vi "NI VeriStand - Close Workspace Window.vi"(8 "error in (no error)":errorcluster, 11 "Project Ref in":T1) -> (0 "error out":errorcluster, 3 "Project Ref out":T1)   [LabVIEW 2020, in "NI_VS Project ExecutionAPI.lvlib"]
doc: "Closes the <B>Workspace</B> window for an NI VeriStand project."
uses:
  <vilib>/NI VeriStand/Execution/Project/NI_VS Project ExecutionAPI.lvlib
  <vilib>/NI VeriStand/Execution/Project/Project Ref.ctl
  NationalInstruments.VeriStand.ClientAPI
  NationalInstruments.VeriStand
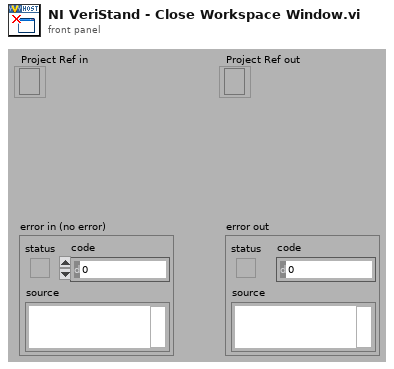
[diagram p1: front panel]
types:
  T1 = typedef "NI_VS Project ExecutionAPI.lvlib/Project Ref.ctl" = refnum<k24>
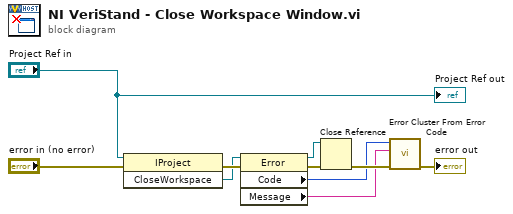
[diagram p0: block diagram]
diagram:
  n1 = invoke class="IProject" method="CloseWorkspace"(reference="Project Ref in", error in="error in (no error)") -> (error out=w8:errorcluster, "CloseWorkspace"=w3:refnum<k24>)  [unwired: 1 in, 1 out]
  n2 = property class="Error"(reference=w3, error in=w8) -> (reference out=w6:refnum<k24>, error out=w7:errorcluster, "Code"=w2:u32, "Message"=w1:string)
  n3 = Close Reference(reference=w6, error in (no error)=w7) -> (error out=w5:errorcluster)
  n4 = call <vilib>:"Error Cluster From Error Code.vi"("error in (no error)"=w5, "error message (\"\")"=w1, "error code (0)"=w2) -> ("error out"=→"error out":errorcluster)  [unwired: 6 in]
  "Project Ref out" <- "Project Ref in"
